vi "Register gRPC Messages.vi"(8 "error in (no error)":errorcluster, 11 "gRPC ID":T1) -> (0 "error out":errorcluster, 3 "gRPC ID Out":T1)   [LabVIEW 2025, in "reflection_client.lvlib"]
uses:
  reflection_client.lvlib
  <vilib>/gRPC/LabVIEW gRPC Library/Shared/grpcId.ctl
  <vilib>/gRPC/LabVIEW gRPC Library/Server API/typeDefs/Message Metadata.ctl
  <vilib>/gRPC/LabVIEW gRPC Library/Server API/typeDefs/Message Element Metadata.ctl
  <vilib>/gRPC/LabVIEW gRPC Library/Server API/typeDefs/Message Element Type.ctl
  <vilib>/gRPC/LabVIEW gRPC Library/Server API/typeDefs/Enum Metadata.ctl
  <vilib>/gRPC/LabVIEW gRPC Library/grpc-lvsupport-release.lvlib
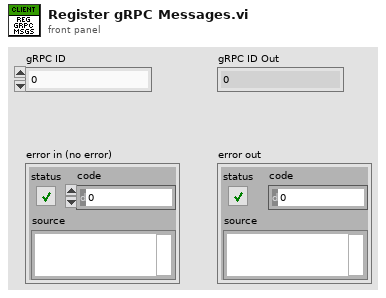
[diagram p1: front panel]
types:
  T1 = typedef "grpc-lvsupport-release.lvlib/grpcId.ctl" = u64
  T2 = typedef "grpc-lvsupport-release.lvlib/Enum Metadata.ctl" = cluster{"Version":i32, "Name":string, "Type Url":string, "Enum Values":string, "Allow Alias":bool}
  T3 = typedef "grpc-lvsupport-release.lvlib/Message Metadata.ctl" = cluster{"Version":i32, "Name":string, "Type Url":string, "Elements":T4[], "Has Oneof":bool}
  T4 = typedef "grpc-lvsupport-release.lvlib/Message Element Metadata.ctl" = cluster{"Field Name":string, "Embedded Message Name":string, "Protobuf Index":i32, "MessageElementType":T5, "Repeated":bool, "Is in Oneof":bool, "Oneof Container Name":string}
  T5 = typedef "grpc-lvsupport-release.lvlib/Message Element Type.ctl" = enum32{"Int32Value", "FloatValue", "DoubleValue", "BoolValue", "StringValue", "MessageValue", "Int64Value", "UInt32Value", "UInt64Value", "EnumValue", "Bytes", "Fixed64", "Fixed32", "SFixed64", "SFixed32", "SInt64", "SInt32"}
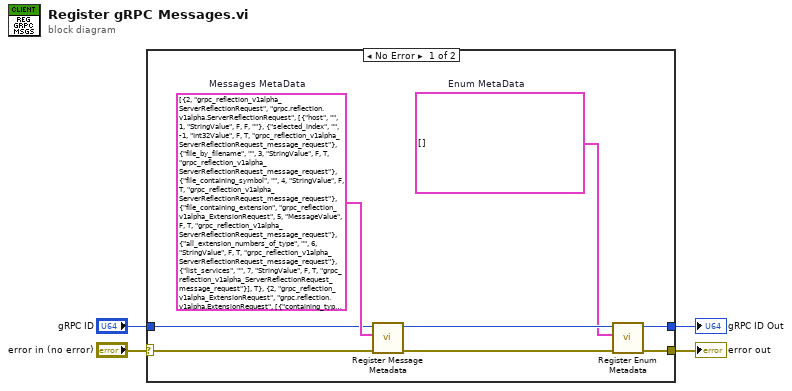
[diagram p0: block diagram]
diagram:
  n1 = case shown="No Error" "error in (no error)" {
    selector: "error in (no error)" -> [w10 w13]
    tunnel: [w9 w12] -> w1
    tunnel: [w6 w13] -> w4
    tunnel: "gRPC ID" -> [w9 w12]
    frame No Error {
      w5 = T2[] []  # Enum MetaData
      w11 = T3[] [{"Version"=2, "Name"="grpc_reflection_v1alpha_ServerReflectionRequest", "Type Url"="grpc.reflection.v1alpha.ServerReflectionRequest", "Elements"=[{"Field Name"="host", "Embedded Message Name"="", "Protobuf Index"=1, "MessageElementType"=enum."StringValue", "Repeated"=FALSE, "Is in Oneof"=FALSE, "Oneof Container Name"=""}, {"Field Name"="selected_index", "Embedded Message Name"="", "Protobuf Index"=-1, "MessageElementType"=enum."Int32Value", "Repeated"=FALSE, "Is in Oneof"=TRUE, "Oneof Container Name"="grpc_reflection_v1alpha_ServerReflectionRequest_message_request"}, {"Field Name"="file_by_filename", "Embedded Message Name"="", "Protobuf Index"=3, "MessageElementType"=enum."StringValue", "Repeated"=FALSE, "Is in Oneof"=TRUE, "Oneof Container Name"="grpc_reflection_v1alpha_ServerReflectionRequest_message_request"}, {"Field Name"="file_containing_symbol", "Embedded Message Name"="", "Protobuf Index"=4, "MessageElementType"=enum."StringValue", "Repeated"=FALSE, "Is in Oneof"=TRUE, "Oneof Container Name"="grpc_reflection_v1alpha_ServerReflectionRequest_message_request"}, {"Field Name"="file_containing_extension", "Embedded Message Name"="grpc_reflection_v1alpha_ExtensionRequest", "Protobuf Index"=5, "MessageElementType"=enum."MessageValue", "Repeated"=FALSE, "Is in Oneof"=TRUE, "Oneof Container Name"="grpc_reflection_v1alpha_ServerReflectionRequest_message_request"}, {"Field Name"="all_extension_numbers_of_type", "Embedded Message Name"="", "Protobuf Index"=6, "MessageElementType"=enum."StringValue", "Repeated"=FALSE, "Is in Oneof"=TRUE, "Oneof Container Name"="grpc_reflection_v1alpha_ServerReflectionRequest_message_request"}, {"Field Name"="list_services", "Embedded Message Name"="", "Protobuf Index"=7, "MessageElementType"=enum."StringValue", "Repeated"=FALSE, "Is in Oneof"=TRUE, "Oneof Container Name"="grpc_reflection_v1alpha_ServerReflectionRequest_message_request"}], "Has Oneof"=TRUE}, {"Version"=2, "Name"="grpc_reflection_v1alpha_ExtensionRequest", "Type Url"="grpc.reflection.v1alpha.ExtensionRequest", "Elements"=[{"Field Name"="containing_type", "Embedded Message Name"="", "Protobuf Index"=1, "MessageElementType"=enum."StringValue", "Repeated"=FALSE, "Is in Oneof"=FALSE, "Oneof Container Name"=""}, {"Field Name"="extension_number", "Embedded Message Name"="", "Protobuf Index"=2, "MessageElementType"=enum."Int32Value", "Repeated"=FALSE, "Is in Oneof"=FALSE, "Oneof Container Name"=""}], "Has Oneof"=FALSE}, {"Version"=2, "Name"="grpc_reflection_v1alpha_ServerReflectionResponse", "Type Url"="grpc.reflection.v1alpha.ServerReflectionResponse", "Elements"=[{"Field Name"="valid_host", "Embedded Message Name"="", "Protobuf Index"=1, "MessageElementType"=enum."StringValue", "Repeated"=FALSE, "Is in Oneof"=FALSE, "Oneof Container Name"=""}, {"Field Name"="original_request", "Embedded Message Name"="grpc_reflection_v1alpha_ServerReflectionRequest", "Protobuf Index"=2, "MessageElementType"=enum."MessageValue", "Repeated"=FALSE, "Is in Oneof"=FALSE, "Oneof Container Name"=""}, {"Field Name"="selected_index", "Embedded Message Name"="", "Protobuf Index"=-1, "MessageElementType"=enum."Int32Value", "Repeated"=FALSE, "Is in Oneof"=TRUE, "Oneof Container Name"="grpc_reflection_v1alpha_ServerReflectionResponse_message_response"}, {"Field Name"="file_descriptor_response", "Embedded Message Name"="grpc_reflection_v1alpha_FileDescriptorResponse", "Protobuf Index"=4, "MessageElementType"=enum."MessageValue", "Repeated"=FALSE, "Is in Oneof"=TRUE, "Oneof Container Name"="grpc_reflection_v1alpha_ServerReflectionResponse_message_response"}, {"Field Name"="all_extension_numbers_response", "Embedded Message Name"="grpc_reflection_v1alpha_ExtensionNumberResponse", "Protobuf Index"=5, "MessageElementType"=enum."MessageValue", "Repeated"=FALSE, "Is in Oneof"=TRUE, "Oneof Container Name"="grpc_reflection_v1alpha_ServerReflectionResponse_message_response"}, {"Field Name"="list_services_response", "Embedded Message Name"="grpc_reflection_v1alpha_ListServiceResponse", "Protobuf Index"=6, "MessageElementType"=enum."MessageValue", "Repeated"=FALSE, "Is in Oneof"=TRUE, "Oneof Container Name"="grpc_reflection_v1alpha_ServerReflectionResponse_message_response"}, {"Field Name"="error_response", "Embedded Message Name"="grpc_reflection_v1alpha_ErrorResponse", "Protobuf Index"=7, "MessageElementType"=enum."MessageValue", "Repeated"=FALSE, "Is in Oneof"=TRUE, "Oneof Container Name"="grpc_reflection_v1alpha_ServerReflectionResponse_message_response"}], "Has Oneof"=TRUE}, {"Version"=2, "Name"="grpc_reflection_v1alpha_FileDescriptorResponse", "Type Url"="grpc.reflection.v1alpha.FileDescriptorResponse", "Elements"=[{"Field Name"="file_descriptor_proto", "Embedded Message Name"="", "Protobuf Index"=1, "MessageElementType"=enum."Bytes", "Repeated"=TRUE, "Is in Oneof"=FALSE, "Oneof Container Name"=""}], "Has Oneof"=FALSE}, {"Version"=2, "Name"="grpc_reflection_v1alpha_ExtensionNumberResponse", "Type Url"="grpc.reflection.v1alpha.ExtensionNumberResponse", "Elements"=[{"Field Name"="base_type_name", "Embedded Message Name"="", "Protobuf Index"=1, "MessageElementType"=enum."StringValue", "Repeated"=FALSE, "Is in Oneof"=FALSE, "Oneof Container Name"=""}, {"Field Name"="extension_number", "Embedded Message Name"="", "Protobuf Index"=2, "MessageElementType"=enum."Int32Value", "Repeated"=TRUE, "Is in Oneof"=FALSE, "Oneof Container Name"=""}], "Has Oneof"=FALSE}, {"Version"=2, "Name"="grpc_reflection_v1alpha_ListServiceResponse", "Type Url"="grpc.reflection.v1alpha.ListServiceResponse", "Elements"=[{"Field Name"="service", "Embedded Message Name"="grpc_reflection_v1alpha_ServiceResponse", "Protobuf Index"=1, "MessageElementType"=enum."MessageValue", "Repeated"=TRUE, "Is in Oneof"=FALSE, "Oneof Container Name"=""}], "Has Oneof"=FALSE}, {"Version"=2, "Name"="grpc_reflection_v1alpha_ServiceResponse", "Type Url"="grpc.reflection.v1alpha.ServiceResponse", "Elements"=[{"Field Name"="name", "Embedded Message Name"="", "Protobuf Index"=1, "MessageElementType"=enum."StringValue", "Repeated"=FALSE, "Is in Oneof"=FALSE, "Oneof Container Name"=""}], "Has Oneof"=FALSE}, {"Version"=2, "Name"="grpc_reflection_v1alpha_ErrorResponse", "Type Url"="grpc.reflection.v1alpha.ErrorResponse", "Elements"=[{"Field Name"="error_code", "Embedded Message Name"="", "Protobuf Index"=1, "MessageElementType"=enum."Int32Value", "Repeated"=FALSE, "Is in Oneof"=FALSE, "Oneof Container Name"=""}, {"Field Name"="error_message", "Embedded Message Name"="", "Protobuf Index"=2, "MessageElementType"=enum."StringValue", "Repeated"=FALSE, "Is in Oneof"=FALSE, "Oneof Container Name"=""}], "Has Oneof"=FALSE}]  # Messages MetaData
      n2 = call <vilib>:"Register Message Metadata.vi"("error in"=w10, "Messages"=w11, "gRPCid in"=w9) -> ("error out"=w7:errorcluster, "gRPCid out"=w8:T1)  [unwired: 7 in]
      n3 = call <vilib>:"Register Enum Metadata.vi"("error in"=w7, "Enum Metadata"=w5, "gRPCid in"=w8) -> ("error out"=w6:errorcluster)  [unwired: 7 in, 1 out]
    }
    frame Error {
    }
  }
  "error out" <- w4
  "gRPC ID Out" <- w1
